vi "armFormulaAngleToEncoderCounts.vi"() -> ()   [LabVIEW 2020]
panel:
  out "y":dbl
  in  "x":dbl
  in  "b":dbl=6.3008
  in  "m":dbl=0.50267
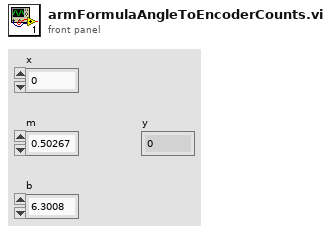
[diagram p1: front panel]
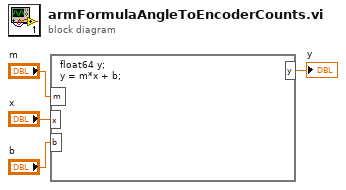
[diagram p0: block diagram]
diagram:
  n1 = formula code="float64 y;\ny = m*x + b;"("m"="m", "x"="x", "b"="b") -> ("y"=→"y":dbl)
